vi "place element in order.vi"(10 "new element":u8, 11 "Array":u8[](array[numeric])) -> (1 "Replace?":bool, 2 "Index":u8)   [LabVIEW 2009]
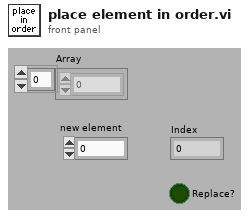
[diagram p1: front panel]
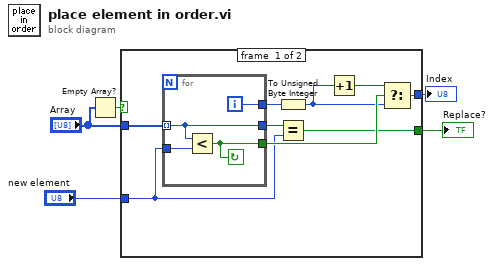
[diagram p0: block diagram]
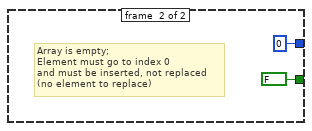
[diagram p2: hidden frame]
diagram:
  n1 = Empty Array?(array="Array") -> (empty?=w2:bool)
  n2 = case shown="True" w2 {
    tunnel: "Array" -> [w14 _]
    tunnel: [w11 u8 0] -> w5
    tunnel: "new element" -> [w9 _]
    tunnel: [w8 FALSE] -> w3
    frame #0 {
      n3 = for {
        tunnel: w9 -> [w18]
        tunnel: w14 -> [w15] mode=indexing
        tunnel: [w17] -> w13
        tunnel: [w16] -> w12
        tunnel: [w15] -> w10
        i -> [w16]
        stop <- w17 continue-if-true
        n4 = Less?(x=w15, y=w18) -> (x < y?=w17:bool)
      }
      n5 = To Unsigned Byte Integer(number=w12) -> (unsigned 8bit integer=w6:u8)
      n6 = Equal?(x=w10, y=w9) -> (x = y?=w8:bool)
      n7 = Increment(x=w6) -> (x+1=w7:u8)
      n8 = Select(t=w7, s=w13, f=w6) -> (s? t:f=w11:u8)
    }
    frame #1 {
      # "Array is empty;\nElement must go to index 0\nand must be inserted, not replaced\n(no element to replace)"
    }
  }
  "Replace?" <- w3
  "Index" <- w5
